vi "Configure Multi Eval Meas Limit PERR.vi"(4 "Peak (50.0)":dbl=50.0 format="%^.3e", 5 "Peak Enabled (Off)":i32(ring) items=["Off", "On", "Value"], 6 "RMS (50.0)":dbl=50.0 format="%^.3e", 7 "RMS Enabled (Off)":i32(ring) items=["Off", "On", "Value"], 8 "error in (no error)":errorcluster, 9 "Modulation (Pi/2-BPSK)":i32(ring) items=["Pi/2-BPSK", "QPSK", "16-QAM", "64-QAM", "256-QAM"], 10 "Instance (1)":T1=1, 11 "VISA resource name":refnum<visa-resource-name>) -> (0 "error out":errorcluster, 3 "VISA resource name out":refnum<visa-resource-name>)   [LabVIEW 2015, in "Rohde&Schwarz CMXP NR FR2 Measurement.lvlib"]
doc: "Defines upper limits for the RMS and peak values of the phase error (PERR) for Pi/2-BPSK.\n\nAttributes:\nRSCMXPNRFR2M_ATTR_MULTI_EVAL_MEASUREMENT_LIMIT_PHBPSK_PERR\nRSCMXPNRFR2M_ATTR_MULTI_EVAL_MEASUREMENT_LIMIT_QPSK_PERR\nRSCMXPNRFR2M_ATTR_MULTI_EVAL_MEASUREMENT_LIMIT_QAM16_PERR\nRSCMXPNRFR2M_ATTR_MULTI_EVAL_MEASUREMENT_LIMIT_QAM64_PERR\nRSCMXPNRFR2M_ATTR_MULTI_EVAL_MEASUREMENT_LIMIT_QAM256_PERR\n\nRemote-control commands:\nCONFigure:NRMMw:MEAS<i>:MEValuation:LIMit:PHBPsk:PERRor\nCONFigure:NRMMw:MEAS<i>:MEValuation:LIMit:QPSK:PERRor\nCONFigure:NRMMw:MEAS<i>:MEValuation:LIMit:QAM<order>:PERRor"
uses:
  <instrlib>/Rohde&Schwarz CMXP NR FR2 Measurement/Rohde&Schwarz CMXP NR FR2 Measurement.lvlib
  <instrlib>/Rohde&Schwarz CMXP NR FR2 Measurement/Private/_Instance.ctl
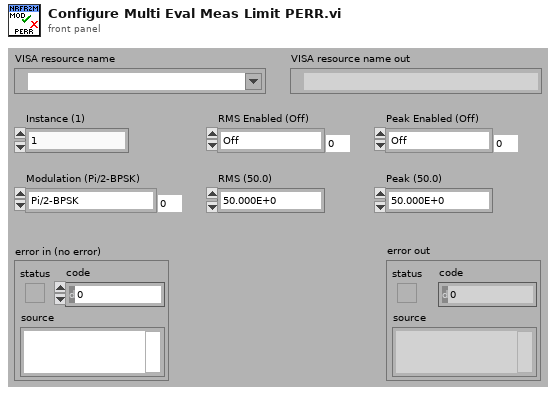
[diagram p1: front panel]
types:
  T1 = typedef "Rohde&Schwarz CMXP NR FR2 Measurement.lvlib/_Instance.ctl" = i32
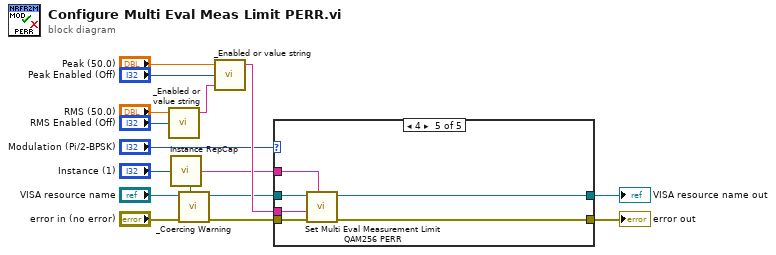
[diagram p0: block diagram]
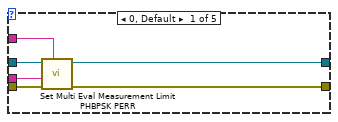
[diagram p2: hidden frame]
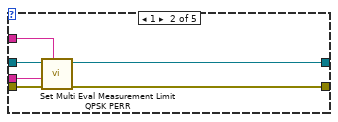
[diagram p3: hidden frame]
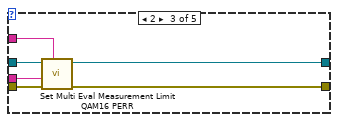
[diagram p4: hidden frame]
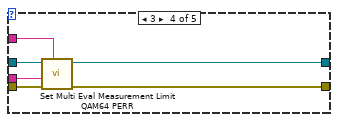
[diagram p5: hidden frame]
diagram:
  n1 = call <instrlib>:"_Enabled or value string.vi"("Enabled or Value"="RMS Enabled (Off)", "Value"="RMS (50.0)") -> ("Resulting String"=w10:string)  [unwired: 3 in]
  n2 = call <instrlib>:"Instance RepCap.vi"("Instance In"="Instance (1)") -> ("In Range?"=w15:bool, "RepCap Identifier Out"=w5:string)  [unwired: 1 in]
  n3 = call <instrlib>:"_Coercing Warning.vi"("In Range?"=w15, "error in (no error)"="error in (no error)", "VISA resource name"="VISA resource name") -> ("error out"=w7:errorcluster, "VISA resource name out"=w6:refnum<visa-resource-name>)  [unwired: 7 in]
  n4 = call <instrlib>:"_Enabled or value string.vi"("Initial String"=w10, "Enabled or Value"="Peak Enabled (Off)", "Value"="Peak (50.0)") -> ("Resulting String"=w8:string)  [unwired: 2 in]
  n5 = case shown="4" "Modulation (Pi/2-BPSK)" {
    tunnel: w8 -> [w17 w23 w29 w35 w41]
    tunnel: w7 -> [w22 w28 w34 w40 w46]
    tunnel: w6 -> [w21 w27 w33 w39 w45]
    tunnel: w5 -> [w20 w26 w32 w38 w44]
    tunnel: [w19 w25 w31 w37 w43] -> w2
    tunnel: [w18 w24 w30 w36 w42] -> w3
    frame 0, Default {
      n6 = call "Set Multi Eval Measurement Limit PHBPSK PERR"("Repeated Capabilities"=w20, "error in (no error)"=w22, "Multi Eval Measurement Limit PHBPSK PERR ()"=w17, "instrument handle"=w21) -> ("error out"=w19:errorcluster, "instrument handle out"=w18:refnum<visa-resource-name>)  [unwired: 6 in]
    }
    frame 1 {
      n7 = call "Set Multi Eval Measurement Limit QPSK PERR"("Repeated Capabilities"=w26, "error in (no error)"=w28, "Multi Eval Measurement Limit QPSK PERR ()"=w23, "instrument handle"=w27) -> ("error out"=w25:errorcluster, "instrument handle out"=w24:refnum<visa-resource-name>)  [unwired: 6 in]
    }
    frame 2 {
      n8 = call "Set Multi Eval Measurement Limit QAM16 PERR"("Repeated Capabilities"=w32, "error in (no error)"=w34, "Multi Eval Measurement Limit QAM16 PERR ()"=w29, "instrument handle"=w33) -> ("error out"=w31:errorcluster, "instrument handle out"=w30:refnum<visa-resource-name>)  [unwired: 6 in]
    }
    frame 3 {
      n9 = call "Set Multi Eval Measurement Limit QAM64 PERR"("Repeated Capabilities"=w38, "error in (no error)"=w40, "Multi Eval Measurement Limit QAM64 PERR ()"=w35, "instrument handle"=w39) -> ("error out"=w37:errorcluster, "instrument handle out"=w36:refnum<visa-resource-name>)  [unwired: 6 in]
    }
    frame 4 {
      n10 = call "Set Multi Eval Measurement Limit QAM256 PERR"("Repeated Capabilities"=w44, "error in (no error)"=w46, "Multi Eval Measurement Limit QAM256 PERR ()"=w41, "instrument handle"=w45) -> ("error out"=w43:errorcluster, "instrument handle out"=w42:refnum<visa-resource-name>)  [unwired: 6 in]
    }
  }
  "error out" <- w2
  "VISA resource name out" <- w3
